vi "Unibot - State Machine Controller.vi"(3 "dt (s)":dbl=-1.0 format="%.3f", 4 "Parameters":T1={"Limit"=10.0, "Control Dead Band"=20.0, "Error Dead Band"=20.0}, 5 "Up Optimal Gain":dbl[](array[numeric])=[-16.4615, -16.2422, -3.1287, -2.0658], 6 "Mode":T2(ring), 7 "Setpoint":dbl(knob) scale=-1.0..1.0, 8 "Enable":bool, 9 "Kill":bool, 10 "PID gains":T3={"proportional gain (Kc)"=1.0, "integral time (Ti, min)"=0.01, "derivative time (Td, min)"=0.0} {"derivative time (Td, min)" format="%.3f"; "integral time (Ti, min)" format="%.3f"; "proportional gain (Kc)" format="%.3f"}, 11 "States":dbl[](array[numeric])=[-0.0012566370614359172, -0.8117875416876026, 0.0, 0.0]) -> (0 "Status":string="Kill", 2 "Control Effort":dbl(knob) scale=-1000.0..1000.0)   [LabVIEW 2012]
uses:
  Unibot - States.ctl
  <vilib>/addons/Control Design/_Implementation/CD State Feedback Controller (Single Output).vi
  <vilib>/addons/control/pid/pid.llb/PID (DBL).vi
  <vilib>/addons/Control Design/_Implementation/NI_CD_Implementation.lvlib
  <vilib>/addons/control/pid/NI_PID_pid.lvlib
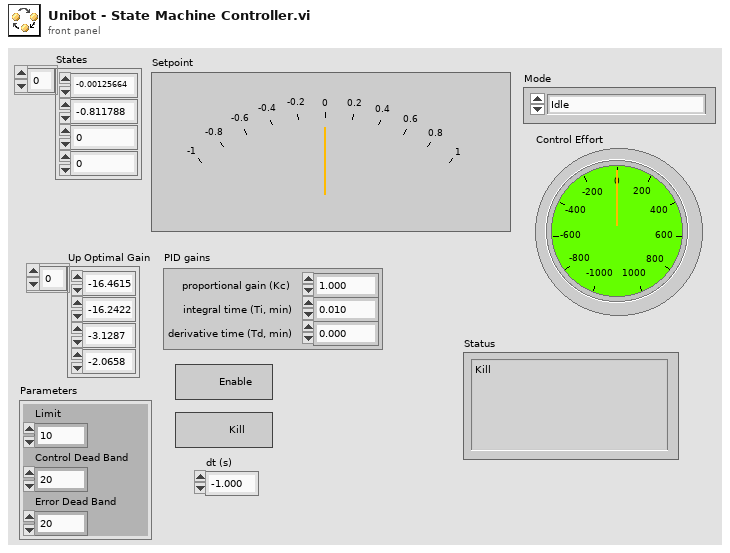
[diagram p1: front panel]
types:
  T1 = cluster{"Limit":dbl, "Control Dead Band":dbl, "Error Dead Band":dbl}
  T2 = enum16{"Idle", "Linear Balance", "Proportional Balance", "PID Balance", "Emergency"}
  T3 = cluster{"proportional gain (Kc)":dbl, "integral time (Ti, min)":dbl, "derivative time (Td, min)":dbl}
  T4 = typedef "Unibot - States.ctl" = enum16{"Idle", "Linear Balance", "Proportional Balance", "PID Balance", "Emergency"}
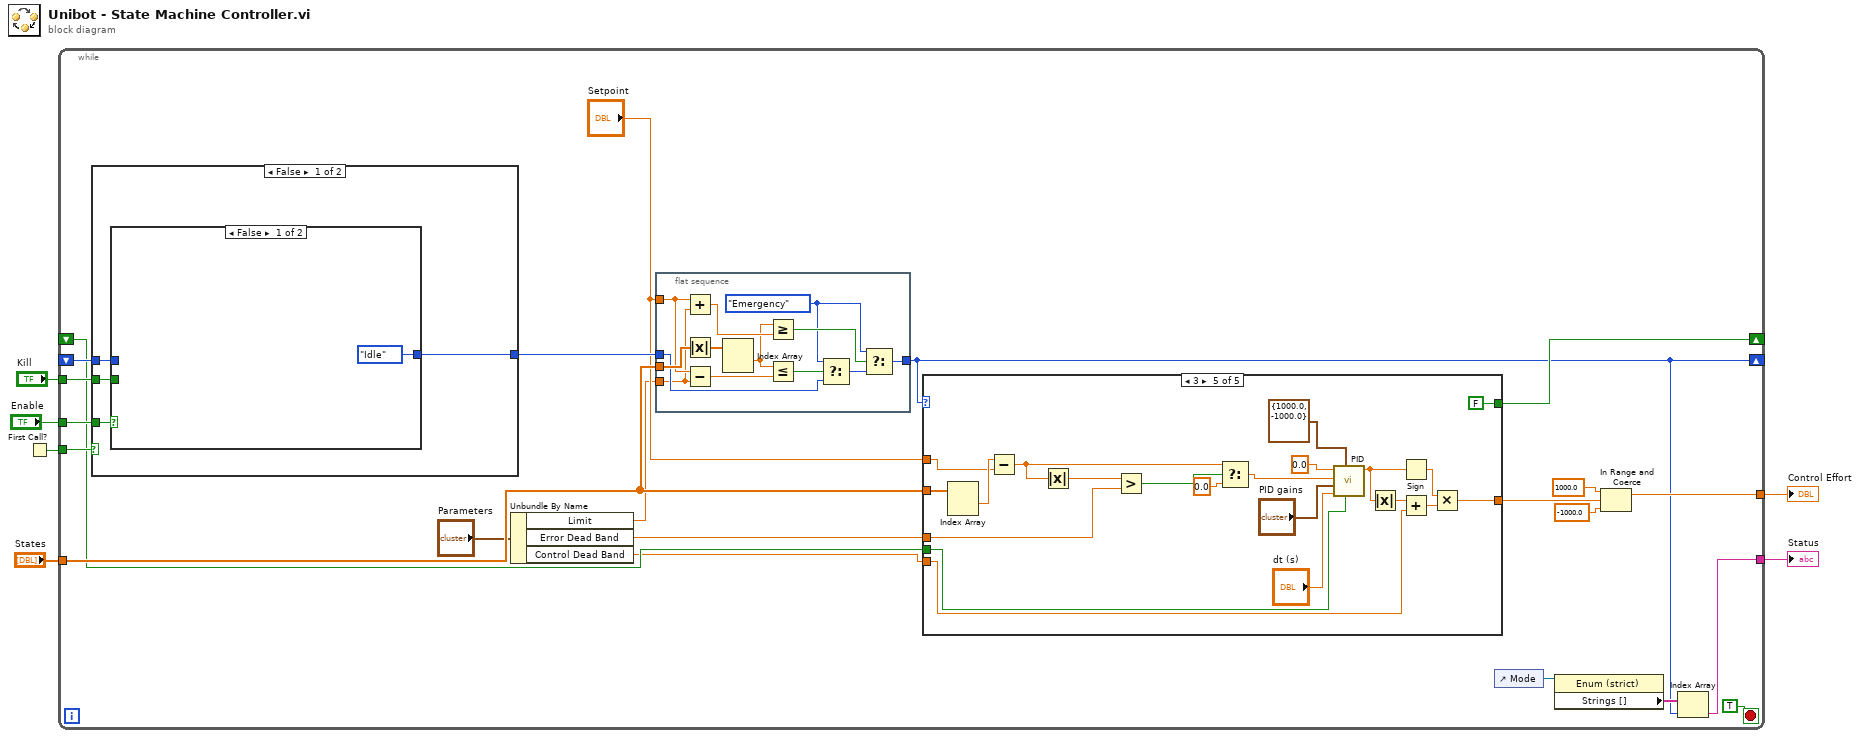
[diagram p0: block diagram]
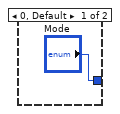
[diagram p3: hidden frame]
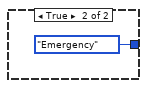
[diagram p4: hidden frame]
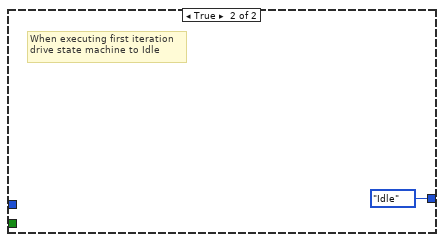
[diagram p5: hidden frame]
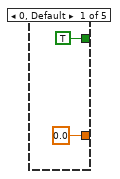
[diagram p6: hidden frame]
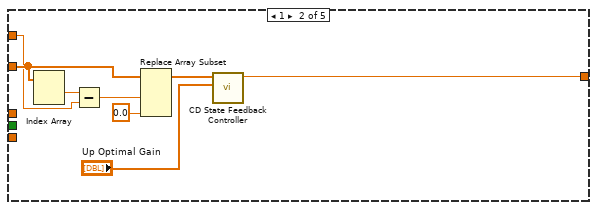
[diagram p7: hidden frame]
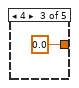
[diagram p8: hidden frame]
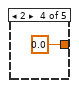
[diagram p9: hidden frame]
diagram:
  n1 = First Call?() -> (First Call?: T/F=w3:bool)
  n2 = while {
    tunnel: "States" -> [w23]
    tunnel: [w20] -> w1
    shift-right: [w12] -> _
    shift-left: _ -> [w26]
    tunnel: [w16] -> w5
    tunnel: "Kill" -> [w27]
    tunnel: w3 -> [w25]
    tunnel: "Enable" -> [w24]
    shift-right: [w14] -> _
    shift-left: _ -> [w15]
    stop <- TRUE stop-if-true
    n3 = case shown="False" w25 {
      tunnel: w27 -> [w45 _]
      tunnel: w26 -> [w44 _]
      tunnel: w24 -> [w43 _]
      tunnel: [w42 Unibot_-_States."Idle" ("Enum")] -> w22
      frame False {
        n4 = case shown="False" w43 {
          tunnel: w45 -> [_ w49]
          tunnel: w44 -> [_ w47]
          tunnel: [Unibot_-_States."Idle" ("Enum") w48] -> w42
          frame False {
          }
          frame True {
            n5 = case shown="False" w49 {
              tunnel: [w50 Unibot_-_States."Emergency" ("Enum")] -> w48
              tunnel: w47 -> [w51 _]
              frame False {
                n6 = case shown="4" w51 {
                  selector: w51 -> [_ w53]
                  tunnel: ["Mode" w53] -> w50
                  frame 0, Default {
                  }
                  frame 4 {
                  }
                }
              }
              frame True {
              }
            }
          }
        }
      }
      frame True {
        # "When executing first iteration\ndrive state machine to Idle"
      }
    }
    n7 = Unbundle By Name("Parameters") -> ("Limit"=w9:dbl, "Error Dead Band"=w8:dbl, "Control Dead Band"=w7:dbl)
    n8 = flat-sequence {
      tunnel: w23 -> [w39]
      tunnel: w22 -> [w32]
      tunnel: [w41] -> w12
      tunnel: "Setpoint" -> [w37]
      tunnel: w9 -> [w29]
      frame #0 {
        w31 = Unibot_-_States."Emergency" ("Enum")
        n9 = Add(x=w37, y=w29) -> (x+y=w35:dbl)
        n10 = Absolute Value(x=w39) -> (abs(x)=w40:dbl[])
        n11 = Subtract(x=w37, y=w29) -> (x-y=w36:dbl)
        n12 = Index Array(array=w40) -> (element #1=w30:dbl)  [unwired: 2 in, 1 out]
        n13 = Greater Or Equal?(x=w30, y=w35) -> (x >= y?=w34:bool)
        n14 = Less Or Equal?(x=w30, y=w36) -> (x <= y?=w38:bool)
        n15 = Select(t=w31, s=w38, f=w32) -> (s? t:f=w33:i32)
        n16 = Select(t=w31, s=w34, f=w33) -> (s? t:f=w41:i32)
      }
    }
    n17 = case shown="3" w12 {
      tunnel: w23 -> [_ w62 _ _ w86]
      tunnel: [0.0 w60 0.0 0.0 ("output") w80] -> w21
      tunnel: "Setpoint" -> [_ w59 _ _ w68]
      tunnel: w15 -> [_ _ _ _ w84]
      tunnel: [TRUE ("Enable") _ _ _ FALSE ("Enable")] -> w14
      tunnel: w7 -> [_ _ _ _ w82]
      tunnel: w8 -> [_ _ _ _ w73]
      frame 0, Default {
      }
      frame 1 {
        n18 = Index Array(array=w62) -> (element #1=w61:dbl)  [unwired: 2 in, 1 out]
        n19 = Subtract(x=w61, y=w59) -> (x-y=w64:dbl)
        n20 = Replace Array Subset(array=w62, new element #1=w64, new element #2=0.0 ("x")) -> (w65:dbl[])  [unwired: 2 in]
        n21 = call-poly <vilib>:"CD State Feedback Controller.vi"("Controller Gain"="Up Optimal Gain", "States"=w65) -> ("Controller Action"=w60:dbl)  [unwired: 1 in, 8 out]
      }
      frame 4 {
      }
      frame 2 {
      }
      frame 3 {
        n22 = Index Array(array=w86) -> (element #1=w69:dbl)  [unwired: 2 in, 1 out]
        n23 = Subtract(x=w69, y=w68) -> (x-y=w70:dbl)
        n24 = Absolute Value(x=w70) -> (abs(x)=w74:dbl)
        n25 = Greater?(x=w74, y=w73) -> (0:w75:bool)
        n26 = Select(t=w70, s=w75, f=0.0) -> (s? t:f=w71:dbl)
        n27 = call-poly <vilib>:"PID.vi"("reinitialize? (F)"=w84, "output range"=cluster{"output high":dbl, "output low":dbl} {"output high"=1000.0, "output low"=-1000.0}, "dt (s)"="dt (s)", "PID gains"="PID gains", "process variable"=w71, "setpoint"=0.0) -> ("output"=w81:dbl)  [unwired: 4 in, 1 out]
        n28 = Absolute Value(x=w81) -> (abs(x)=w79:dbl)
        n29 = Sign(1:w81) -> (0:w78:dbl)
        n30 = Add(x=w79, y=w82) -> (x+y=w77:dbl)
        n31 = Multiply(x=w78, y=w77) -> (x*y=w80:dbl)
      }
    }
    n32 = control-ref of="Mode"() -> (w13:refnum<vi>)
    n33 = property class="Enum (strict)"(reference=w13) -> ("Strings []"=w17:string[])  [unwired: 1 in, 2 out]
    n34 = In Range and Coerce(upper limit=1000.0, x=w21, lower limit=-1000.0) -> (coerced(x)=w20:dbl)  [unwired: 1 out]
    n35 = Index Array(array=w17, index=w12) -> (element=w16:string)
  }
  "Control Effort" <- w1
  "Status" <- w5
